vi "init.vi"(0 "hid_info":T2, 11 "error in (no error)":errorcluster) -> (3 "str_serial":string, 4 "hid_info out":T2, 6 "fw_info out":T1, 8 "str_mfr":string, 10 "str_product":string, 13 "return type":u64, 14 "str_index_1":string, 15 "error out":errorcluster)   [LabVIEW 2017, in "buddy.lvlib"]
doc: "EXPORT hid_device* buddy_init(buddy_hid_info_t *hid_info, firmware_info_t *fw_info);"
uses:
  buddy.lvlib
  <vilib>/Utility/importsl/GetValueByPointer/datatype.ctl
  <vilib>/Utility/importsl/GetValueByPointer/GetValueByPointer.xnode
  buddy_x64.dll
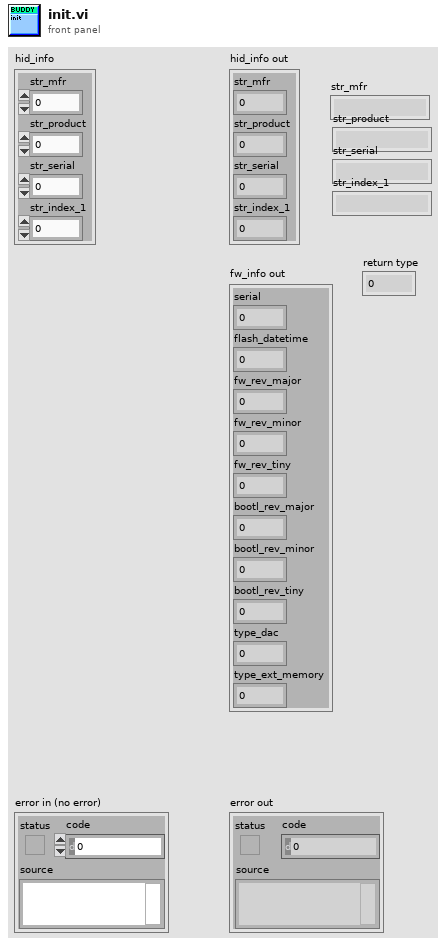
[diagram p1: front panel]
types:
  T1 = cluster{"serial":u32, "flash_datetime":u32, "fw_rev_major":u8, "fw_rev_minor":u8, "fw_rev_tiny":u8, "bootl_rev_major":u8, "bootl_rev_minor":u8, "bootl_rev_tiny":u8, "type_dac":u8, "type_ext_memory":u8}
  T2 = cluster{"str_mfr":u64, "str_product":u64, "str_serial":u64, "str_index_1":u64}
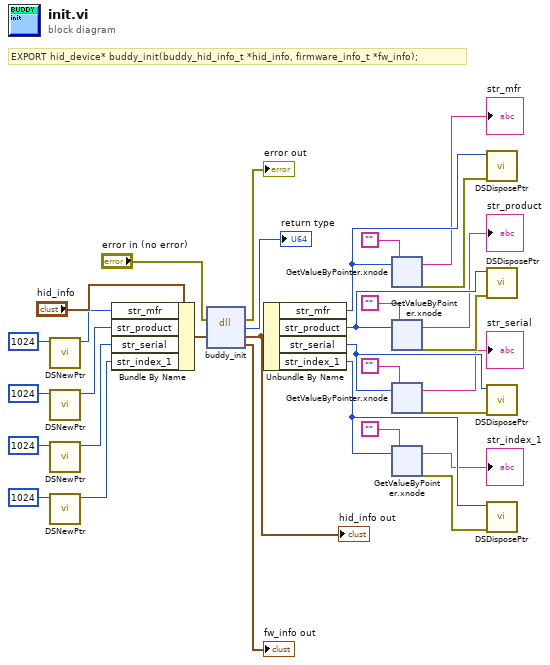
[diagram p0: block diagram]
diagram:
  # "EXPORT hid_device* buddy_init(buddy_hid_info_t *hid_info, firmware_info_t *fw_info);"
  n1 = call <vilib>:"DSNewPtr.vi"("Size"=u64 1024) -> ("Pointer"=w26:u64)  [unwired: 9 in, 1 out]
  n2 = call <vilib>:"DSNewPtr.vi"("Size"=u64 1024) -> ("Pointer"=w24:u64)  [unwired: 9 in, 1 out]
  n3 = call <vilib>:"DSNewPtr.vi"("Size"=u64 1024) -> ("Pointer"=w23:u64)  [unwired: 9 in, 1 out]
  n4 = call <vilib>:"DSNewPtr.vi"("Size"=u64 1024) -> ("Pointer"=w22:u64)  [unwired: 9 in, 1 out]
  n5 = Bundle By Name(cluster="hid_info", "str_mfr"=w26, "str_product"=w24, "str_serial"=w23, "str_index_1"=w22) -> (w25:T2)
  n6 = dll-call lib="C:/Users/shraken/shraken_code/usbhid_buddy/lib/libbuddy/bindings/labview/utility_vi/buddy_x64.dll" fn="buddy_init"(error in="error in (no error)", "hid_info"=w25) -> (error out=→"error out":errorcluster, "return type"=→"return type":u64, "hid_info"=w2:T2, "fw_info out"=→"fw_info out":T1)  [unwired: 3 in, 1 out]
  "hid_info out" <- w2
  n7 = Unbundle By Name(w2) -> ("str_mfr"=w20:u64, "str_product"=w16:u64, "str_serial"=w12:u64, "str_index_1"=w8:u64)
  n8 = xnode "GetValueByPointer.xnode"("Pointer"=w20, "InputType"="") -> ("Output"=→"str_mfr":string, "ErrorOut"=w21:errorcluster)  [unwired: 2 in]
  n9 = xnode "GetValueByPointer.xnode"("Pointer"=w16, "InputType"="") -> ("Output"=→"str_product":string, "ErrorOut"=w17:errorcluster)  [unwired: 2 in]
  n10 = xnode "GetValueByPointer.xnode"("Pointer"=w12, "InputType"="") -> ("Output"=→"str_serial":string, "ErrorOut"=w13:errorcluster)  [unwired: 2 in]
  n11 = xnode "GetValueByPointer.xnode"("Pointer"=w8, "InputType"="") -> ("Output"=→"str_index_1":string, "ErrorOut"=w9:errorcluster)  [unwired: 2 in]
  n12 = call <vilib>:"DSDisposePtr.vi"("error in (no error)"=w21, "Pointer"=w20) -> ()  [unwired: 9 in, 1 out]
  n13 = call <vilib>:"DSDisposePtr.vi"("error in (no error)"=w17, "Pointer"=w16) -> ()  [unwired: 9 in, 1 out]
  n14 = call <vilib>:"DSDisposePtr.vi"("error in (no error)"=w13, "Pointer"=w12) -> ()  [unwired: 9 in, 1 out]
  n15 = call <vilib>:"DSDisposePtr.vi"("error in (no error)"=w9, "Pointer"=w8) -> ()  [unwired: 9 in, 1 out]
